vi "WriteDataVariant.vi"(8 "error in (no error)":errorcluster, 10 "DataVariant":variant, 11 "Singleton.lvclass In":refnum<class "Singleton.lvclass">) -> (0 "error out":errorcluster, 3 "SingletonDVR Out":refnum<data-value>)   [LabVIEW 2014, in "Singleton.lvclass"]
uses:
  Singleton.lvclass
  Singleton.lvclass/Singleton.ctl
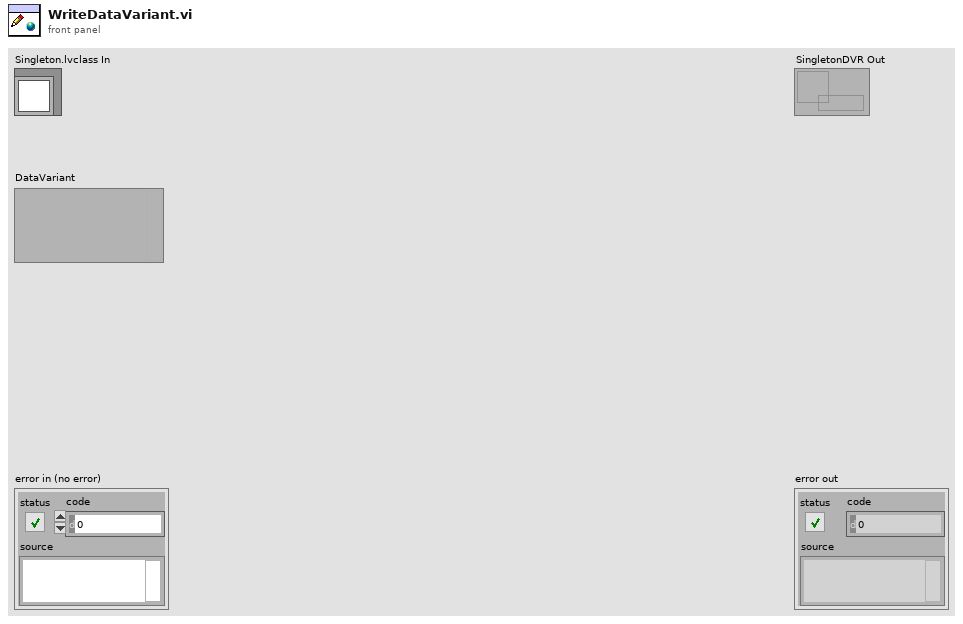
[diagram p1: front panel]
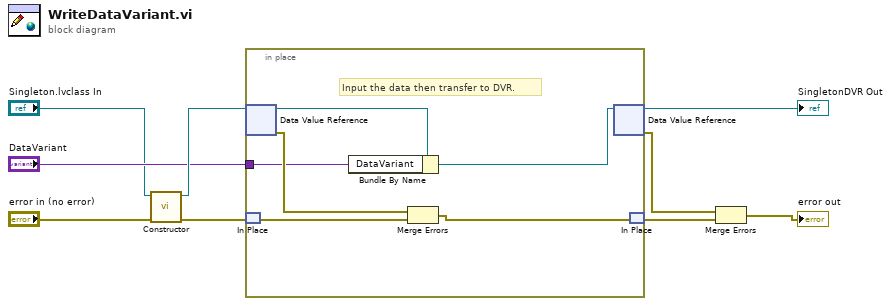
[diagram p0: block diagram]
diagram:
  n1 = call "Constructor.vi"("error in (no error)"="error in (no error)", "Singleton.lvclass In"="Singleton.lvclass In") -> ("error out"=w7:errorcluster, "SingletonDVR Out"=w8:refnum<data-value>)  [unwired: 8 in]
  n2 = in-place {
    in-place-border: "DataVariant" -> [w11]
    # "Input the data then transfer to DVR."
    n3 = in-place-dvr #1(w8) -> (w12:refnum<class "Singleton.lvclass">, w13:errorcluster)
    n4 = in-place-match #2(w7) -> (w15:errorcluster)
    n5 = Bundle By Name(cluster=w12, "DataVariant"=w11) -> (w10:refnum<class "Singleton.lvclass">)
    n6 = Merge Errors(w13, w15) -> (w14:errorcluster)
    n7 = in-place-dvr #1(w10) -> (→"SingletonDVR Out":refnum<data-value>, w4:errorcluster)
    n8 = in-place-match #2(w14) -> (w5:errorcluster)
  }
  n9 = Merge Errors(w4, w5) -> (→"error out":errorcluster)
